vi "Set Enabled States on Multiple Controls.vi"(1 "Enable?":bool, 2 "Control Refnums":refnum<vi>[](array[refnum])) -> ()   [LabVIEW 2016]
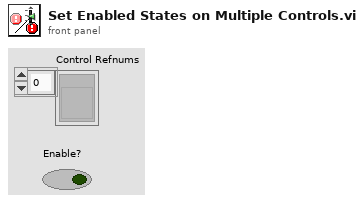
[diagram p1: front panel]
types:
  T1 = enum8{"Enabled", "Disabled", "Disabled and Grayed Out"}
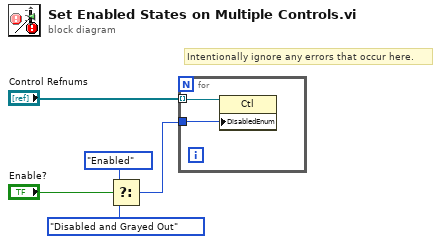
[diagram p0: block diagram]
diagram:
  # "Intentionally ignore any errors that occur here."
  n1 = Select(t=T1."Enabled" ("Disabled"), s="Enable?", f=T1."Disabled and Grayed Out" ("Disabled")) -> (s? t:f=w3:T1)
  n2 = for {
    tunnel: "Control Refnums" -> [w7] mode=indexing
    tunnel: w3 -> [w6]
    n3 = property class="Ctl"(reference=w7, "DisabledEnum"=w6) -> ()  [unwired: 1 in, 2 out]
  }
